vi "VER_SCALE_SETTING.vi"(0 "VER RANGE":string, 1 "VOLTS/DIV":enum32{"CH 1", "CH 2", "CH 3", "CH 4"}(radio), 2 "VISA resource name":refnum<visa-resource-name>="GPIB0::1::INSTR") -> ()   [LabVIEW 2011]
panel:
  # "TDS2014B"
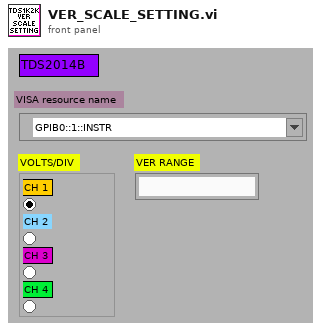
[diagram p1: front panel]
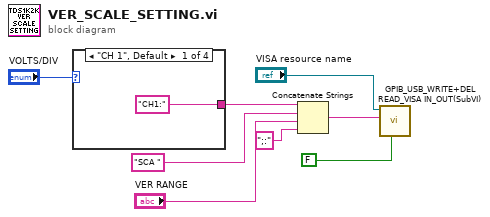
[diagram p0: block diagram]
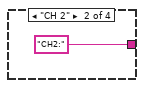
[diagram p2: hidden frame]
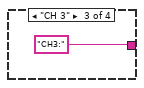
[diagram p3: hidden frame]
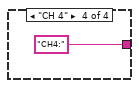
[diagram p4: hidden frame]
diagram:
  n1 = case shown="\"CH 1\", Default" "VOLTS/DIV" {
    tunnel: ["CH1:" "CH2:" "CH3:" "CH4:"] -> w6
    frame "CH 1", Default {
    }
    frame "CH 2" {
    }
    frame "CH 3" {
    }
    frame "CH 4" {
    }
  }
  n2 = Concatenate Strings(w6, "SCA ", "VER RANGE", ";:") -> (w2:string)
  n3 = call "GPIB_USB_WRITE+DEL READ_VISA IN_OUT(SubVI).vi"("VISA resource IN"="VISA resource name", "GPIB/USB WRITE"=w2, 4:FALSE ("READ GPIB")) -> ()  [unwired: 3 in, 3 out]
